vi "Simulated_Field_Open_Field_Info_File.vi"() -> (0 "error out":errorcluster, 3 "Refnum out":T1)   [LabVIEW 2019, in "Simulated_Field.lvlib"]
uses:
  <vilib>/Utility/config.llb/Config Data RefNum.ctl
  Simulated_Field.lvlib
  <vilib>/Utility/config.llb/NI_LVConfig.lvlib
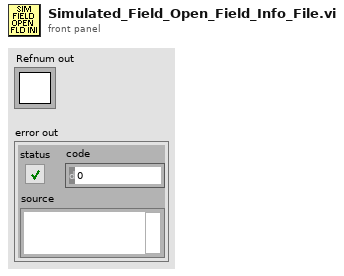
[diagram p1: front panel]
types:
  T1 = typedef "NI_LVConfig.lvlib/Config Data RefNum.ctl" = refnum<k1>
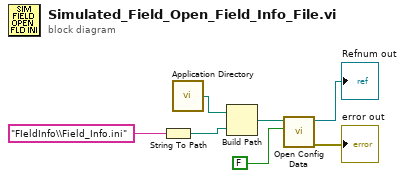
[diagram p0: block diagram]
diagram:
  n1 = String To Path(string="FIeldInfo\\Field_Info.ini") -> (path=w6:path)
  n2 = call <vilib>:"Application Directory.vi"() -> ("Application Directory"=w3:path)
  n3 = Build Path(base path=w3, name or relative path=w6) -> (appended path=w4:path)
  n4 = call <vilib>:"Open Config Data.vi"("create file if necessary (T)"=FALSE, "configuration file path"=w4) -> ("error out"=→"error out":errorcluster, "refnum"=→"Refnum out":T1)  [unwired: 7 in, 1 out]
